vi "Mouse Up Test.vi"() -> ()   [LabVIEW 2021]
panel:
  out "initialized array":timestamp[](array[timestamp])
  in  "dimension size":i32
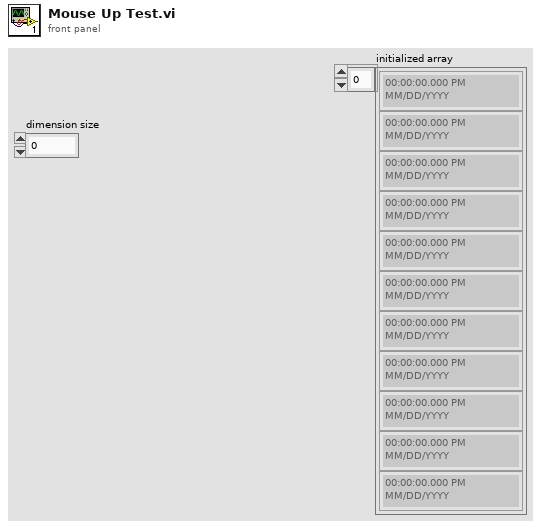
[diagram p1: front panel]
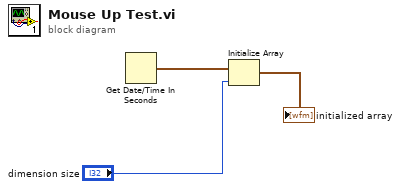
[diagram p0: block diagram]
diagram:
  n1 = Get Date/Time In Seconds() -> (seconds since 1Jan1904=w3:timestamp)
  n2 = Initialize Array(w3, "dimension size") -> (→"initialized array":timestamp[])
